vi "Lone Spikes chopper.vi"(4 "Spikes Array In":cluster{"Index":i32, "max value":dbl}[](array[cluster]), 7 "C Trace":dbl[](array[numeric])) -> (0 "Spikes Array Out":cluster{"Index":i32, "max value":dbl}[](array[cluster]), 1 "No of Removed spikes":i32, 2 "Threshold Value":dbl, 3 "Filtered Time Trace":dbl[](array[numeric]))   [LabVIEW 2022 SP3]
uses:
  <vilib>/Analysis/NI_AALBase.lvlib
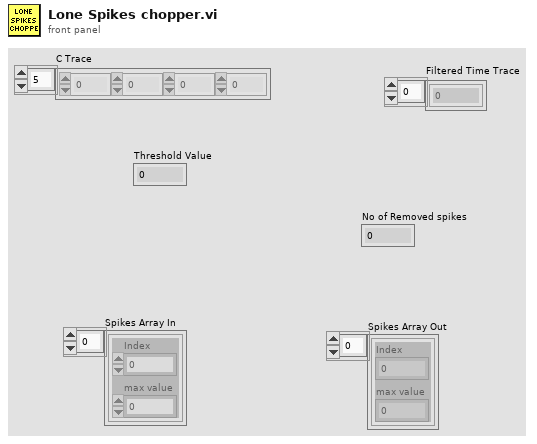
[diagram p1: front panel]
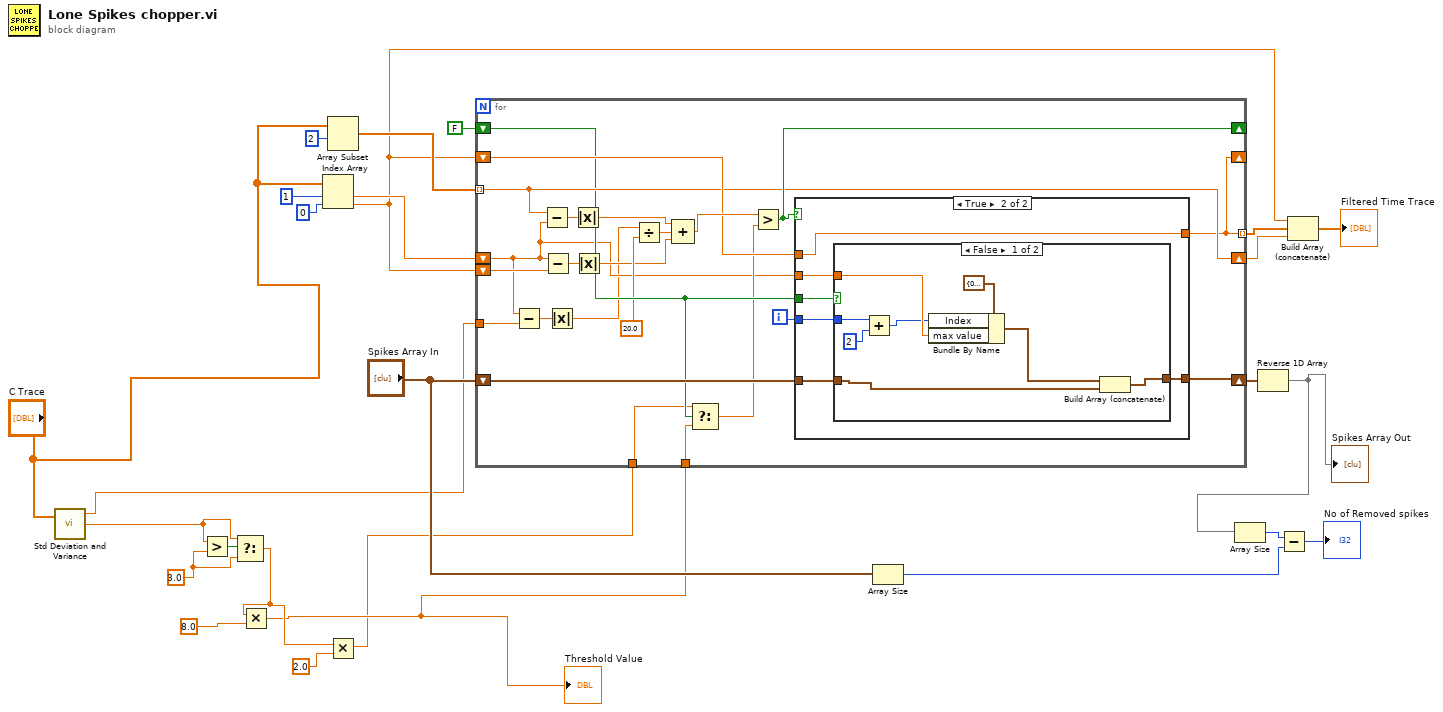
[diagram p0: block diagram]
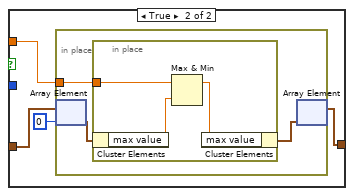
[diagram p3: hidden frame]
diagram:
  w20 = 3.0 ("y")
  n1 = call <vilib>:"Std Deviation and Variance.vi"("X"="C Trace") -> ("mean"=w3:dbl, "standard deviation"=w19:dbl)  [unwired: 1 in, 1 out]
  n2 = Greater?(x=w19, y=w20) -> (0:w21:bool)
  n3 = Select(t=w19, s=w21, f=w20) -> (s? t:f=w10:dbl)
  n4 = Multiply(x=w10, y=8.0) -> (x*y=w2:dbl)
  "Threshold Value" <- w2
  n5 = Index Array(array="C Trace", index #1=1 ("index"), index #2=0 ("index")) -> (element #1=w14:dbl, element #2=w11:dbl)
  n6 = Array Subset(array="C Trace", index=2) -> (w15:dbl[])  [unwired: 1 in]
  n7 = Multiply(x=w10, y=2.0) -> (x*y=w1:dbl)
  n8 = for {
    tunnel: [w39] -> w13 mode=indexing
    tunnel: w15 -> [w40] mode=indexing
    shift-right: [w40] -> w12
    shift-left: w14 -> [w29]
    shift-right: [w49] -> _
    shift-left: FALSE -> [w38]
    shift-right: [w46] -> w7
    shift-left: "Spikes Array In" -> [w47]
    shift-left: w11 -> [w45]
    shift-right: [w39] -> _
    shift-left: w11 -> [w41]
    tunnel: w1 -> [w37]
    tunnel: w2 -> [w36]
    tunnel: w3 -> [w30]
    i -> [w48]
    n9 = Subtract(x=w29, y=w30) -> (x-y=w28:dbl)
    n10 = Subtract(x=w40, y=w29) -> (x-y=w43:dbl)
    n11 = Subtract(x=w29, y=w45) -> (x-y=w44:dbl)
    n12 = Absolute Value(x=w28) -> (abs(x)=w27:dbl)
    n13 = Absolute Value(x=w43) -> (abs(x)=w31:dbl)
    n14 = Absolute Value(x=w44) -> (abs(x)=w32:dbl)
    n15 = Divide(x=w27, y=20.0) -> (x/y=w34:dbl)
    n16 = Compound Arithmetic op=ADD(w31, w34, w32) -> (w42:dbl)
    n17 = Select(t=w37, s=w38, f=w36) -> (s? t:f=w35:dbl)
    n18 = Greater?(x=w42, y=w35) -> (0:w49:bool)
    n19 = case shown="True" w49 {
      tunnel: [w51 w57] -> w39
      tunnel: w29 -> [w51 w54]
      tunnel: w41 -> [_ w57]
      tunnel: w38 -> [_ w56]
      tunnel: w48 -> [_ w55]
      tunnel: w47 -> [w50 w53]
      tunnel: [w50 w52] -> w46
      frame False {
      }
      frame True {
        n20 = case shown="False" w56 {
          tunnel: w55 -> [w60 _]
          tunnel: w54 -> [w64 w67]
          tunnel: w53 -> [w61 w69]
          tunnel: [w63 w66] -> w52
          frame False {
            n21 = Add(x=w60, y=2) -> (x+y=w59:i32)
            n22 = Bundle By Name(cluster=cluster{"Index":i32, "max value":dbl} {"Index"=0, "max value"=0.0} ("output cluster"), "Index"=w59, "max value"=w64) -> (w62:cluster{"Index":i32, "max value":dbl})
            n23 = Build Array (concatenate)(w62, w61) -> (w63:cluster{"Index":i32, "max value":dbl}[])
          }
          frame True {
            n24 = in-place {
              in-place-border: w67 -> [w71]
              n25 = in-place-array #1(w69, 0) -> (w72:cluster{"Index":i32, "max value":dbl})
              n26 = in-place {
                in-place-border: w71 -> [w74]
                n27 = in-place-cluster #2(w72) -> ("max value"=w75:dbl)
                n28 = Max & Min(x=w74, y=w75) -> (max(x,y)=w73:dbl)  [unwired: 1 out]
                n29 = in-place-cluster #2("max value"=w73) -> (w70:cluster{"Index":i32, "max value":dbl})
              }
              n30 = in-place-array #1(w70) -> (w66:cluster{"Index":i32, "max value":dbl}[])  [unwired: 1 out]
            }
          }
        }
      }
    }
  }
  n31 = Array Size(array="Spikes Array In") -> (size(s)=w24:i32)
  n32 = Reverse 1D Array(array=w7) -> (reversed array=w6:cluster{"Index":i32, "max value":dbl}[])
  "Spikes Array Out" <- w6
  n33 = Array Size(array=w6) -> (size(s)=w25:i32)
  n34 = Subtract(x=w25, y=w24) -> (x-y=→"No of Removed spikes":i32)
  n35 = Build Array (concatenate)(w11, w13, w12) -> (→"Filtered Time Trace":dbl[])
